vi "SP7_Kommunikation.vi"(8 "Fehler in":T1, 11 "Cluster in":T2={"Initialisierung"={"Online?"=FALSE, "Grundpfad"=path "", "Kamera Oben"="", "IP-Adresse Flüssiglinse"="", "Flüssiglinse"=refnum, "Kamera Unten"="", "IP-Adresse SPS"="", "SPS-Verbindung"={"TCP Connection Ref"=refnum, "IP address"="", "timeout ms"=5000, "Connected?"=FALSE, "PLC Type"=enum."S7 1200", "Rack S7 400"=0, "Slot S7 400"=0, "PDU Size"=0, "connection semaphore"=refnum}, "IP-Adresse Lichtgitter"="", "Lichtgitter"=refnum, "Skalierungsfaktor"=0.0, "Bilder Oben"=[], "Bild Unten"=refnum, "Bild Ausschnitt Unten"=refnum}, "Einstellungen"={"Gesamtablauf gestartet"=FALSE, "i. O. Bilder speichern"=FALSE, "Bildspeicherung Offline"=FALSE, "Ausgewähltes Offline-Datum"="", "Ausgewähltes Offline-Teil"="", "Speicherpfad Bilder"=path ""}, "Artikeldaten"={"Artikelnummer"="", "Fertigungsauftrag"="", "Muster ISO"=refnum, "Belichtungszeit Referenzmarken"=0.0, "Fokus Referenzmarken"=0.0, "Belichtungszeit ISO"=0.0, "Fokus ISO"=0.0, "Belichtungszeit Unten"=0.0, "Kontaktanzahl"=0, "Aktueller Kontakt"=0, "Kontaktposition"={"x"=0.0, "y"=0.0}, "Winkel ISO"=0.0, "ISO-Muster nicht vorhanden"=FALSE}, "Werte Kamera Oben"={"Koordinatensystem"={"Punkt x-Achse"={"X"=0.0, "Y"=0.0}, "Ursprung"={"X"=0.0, "Y"=0.0}, "Punkt y-Achse"={"X"=0.0, "Y"=0.0}}, "Position Kontakt"={"x"=0.0, "y"=0.0}, "Winkel Kontakt"=0.0}, "Werte Kamera Unten"={"Prüfung Unten n. i. O."=FALSE}, "Werte Lichtgitter"={"Messwerte Referenzmarken"=[], "Mittelpunkt Referenzmarken"={"x"=0.0, "y"=0.0}, "Messwerte Kontakt"=[], "Offset"={"x"=0.0, "y"=0.0}}, "Rückmeldungen"={"Koordinaten ermittelt"=FALSE, "Vermessung Lichtgitter fertig"=FALSE, "Nachkontrolle Kamera Unten fertig"=FALSE}, "Fehler"={"Referenzen nicht gefunden"=FALSE, "Kontakt nicht gefunden"=FALSE, "Referenzen nicht in Lichtgitter"=FALSE, "Kontakt zu groß"=FALSE, "Kontakt zu klein"=FALSE}, "Statistik"={"Statistiken"=[]}, "Timer"={"Timer Start Position"=0, "Timer Start Lichtgitter"=0, "Timer Start Kamera Unten"=0}}) -> (0 "error out":errorcluster)   [LabVIEW 2024]
doc: "Schreibt & liest alle Variablen der SPS."
uses:
  Cluster.ctl
  Kontaktmontagemodul.exe/1abvi3w/vi.lib/userDefined/High Color/IMAQdx.ctl
  Kontaktmontagemodul.exe/1abvi3w/vi.lib/DATA AHEAD/SP7/typedefs/S7 Connection.ctl
  Kontaktmontagemodul.exe/1abvi3w/vi.lib/DATA AHEAD/SP7/typedefs/PLC Type.ctl
  Kontaktmontagemodul.exe/1abvi3w/vi.lib/vision/Image Controls.llb/IMAQ Image.ctl
  Koordinatensystem.ctl
  Statistik.ctl
  Cluster_Fehler_Initialisierung.ctl
  Globale Variablen.vi
  Kontaktmontagemodul.exe/1abvi3w/vi.lib/DATA AHEAD/SP7/SP7.lvlib
panel:
  out "Druchlaufzeit (ms)":u32
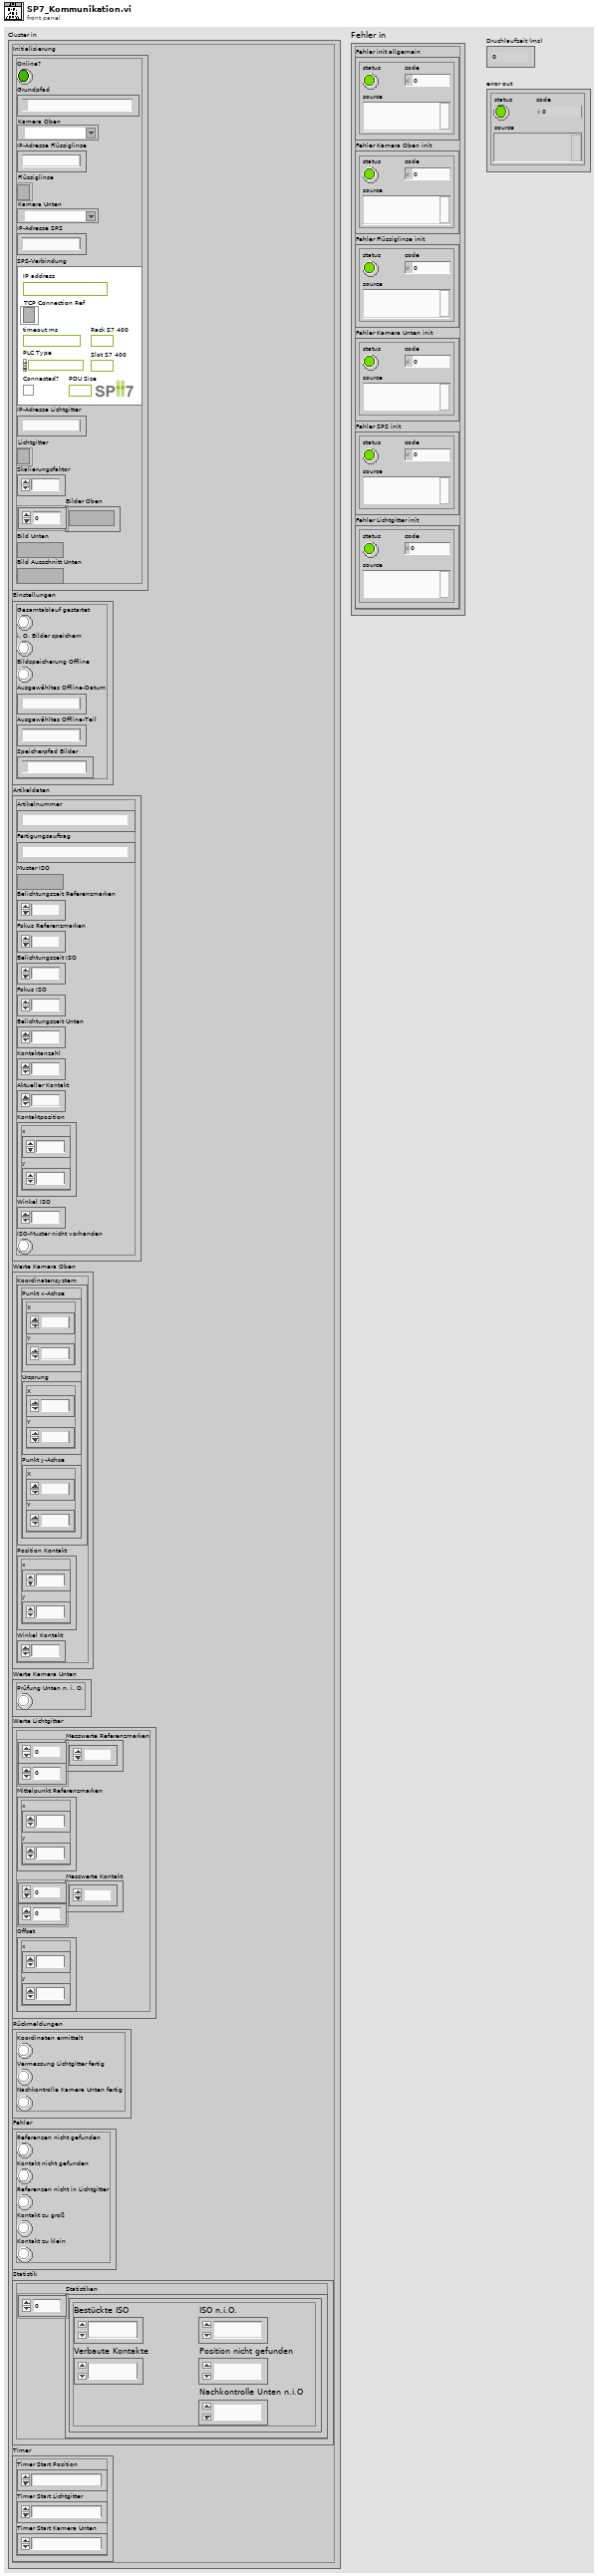
[diagram p1: front panel]
types:
  T1 = typedef "Cluster_Fehler_Initialisierung.ctl" = cluster{"Fehler init allgemein":errorcluster, "Fehler Kamera Oben init":errorcluster, "Fehler Flüssiglinse init":errorcluster, "Fehler Kamera Unten init":errorcluster, "Fehler SPS init":errorcluster, "Fehler Lichtgitter init":errorcluster}
  T2 = typedef "Cluster.ctl" = cluster{"Initialisierung":cluster{"Online?":bool, "Grundpfad":path, "Kamera Oben":T3, "IP-Adresse Flüssiglinse":string, "Flüssiglinse":refnum<k5>, "Kamera Unten":T3, "IP-Adresse SPS":string, "SPS-Verbindung":T4, "IP-Adresse Lichtgitter":string, "Lichtgitter":refnum<k5>, "Skalierungsfaktor":dbl, "Bilder Oben":T7[], "Bild Unten":T7, "Bild Ausschnitt Unten":T7}, "Einstellungen":cluster{"Gesamtablauf gestartet":bool, "i. O. Bilder speichern":bool, "Bildspeicherung Offline":bool, "Ausgewähltes Offline-Datum":string, "Ausgewähltes Offline-Teil":string, "Speicherpfad Bilder":path}, "Artikeldaten":cluster{"Artikelnummer":string, "Fertigungsauftrag":string, "Muster ISO":T7, "Belichtungszeit Referenzmarken":dbl, "Fokus Referenzmarken":dbl, "Belichtungszeit ISO":dbl, "Fokus ISO":dbl, "Belichtungszeit Unten":dbl, "Kontaktanzahl":u32, "Aktueller Kontakt":i16, "Kontaktposition":cluster{"x":sgl, "y":sgl}, "Winkel ISO":sgl, "ISO-Muster nicht vorhanden":bool}, "Werte Kamera Oben":cluster{"Koordinatensystem":T8, "Position Kontakt":cluster{"x":dbl, "y":dbl}, "Winkel Kontakt":dbl}, "Werte Kamera Unten":cluster{"Prüfung Unten n. i. O.":bool}, "Werte Lichtgitter":cluster{"Messwerte Referenzmarken":dbl[][], "Mittelpunkt Referenzmarken":cluster{"x":dbl, "y":dbl}, "Messwerte Kontakt":dbl[][], "Offset":cluster{"x":dbl, "y":dbl}}, "Rückmeldungen":cluster{"Koordinaten ermittelt":bool, "Vermessung Lichtgitter fertig":bool, "Nachkontrolle Kamera Unten fertig":bool}, "Fehler":cluster{"Referenzen nicht gefunden":bool, "Kontakt nicht gefunden":bool, "Referenzen nicht in Lichtgitter":bool, "Kontakt zu groß":bool, "Kontakt zu klein":bool}, "Statistik":cluster{"Statistiken":T9[]}, "Timer":cluster{"Timer Start Position":u32, "Timer Start Lichtgitter":u32, "Timer Start Kamera Unten":u32}}
  T3 = typedef "IMAQdx.ctl" = refnum<k21>
  T4 = typedef "SP7.lvlib/S7 Connection.ctl" = cluster{"TCP Connection Ref":refnum<k5>, "IP address":string, "timeout ms":i32, "Connected?":bool, "PLC Type":T5, "Rack S7 400":u8, "Slot S7 400":u8, "PDU Size":u16, "connection semaphore":T6}
  T5 = typedef "SP7.lvlib/PLC Type.ctl" = enum16{"S7 200", "S7 300/400", "S7 1200", "S7 1500", "LOGO!8"}
  T6 = typedef "Semaphore RefNum" = refnum<k1>
  T7 = typedef "IMAQ Image.ctl" = refnum<image>
  T8 = typedef "Koordinatensystem.ctl" = cluster{"Punkt x-Achse":cluster{"X":sgl, "Y":sgl}, "Ursprung":cluster{"X":sgl, "Y":sgl}, "Punkt y-Achse":cluster{"X":sgl, "Y":sgl}}
  T9 = typedef "Statistik.ctl" = cluster{"Bestückte ISO":u32, "Verbaute Kontakte":u32, "ISO n.i.O.":u32, "Nachkontrolle Unten n.i.O":u32, "Position nicht gefunden":u32}
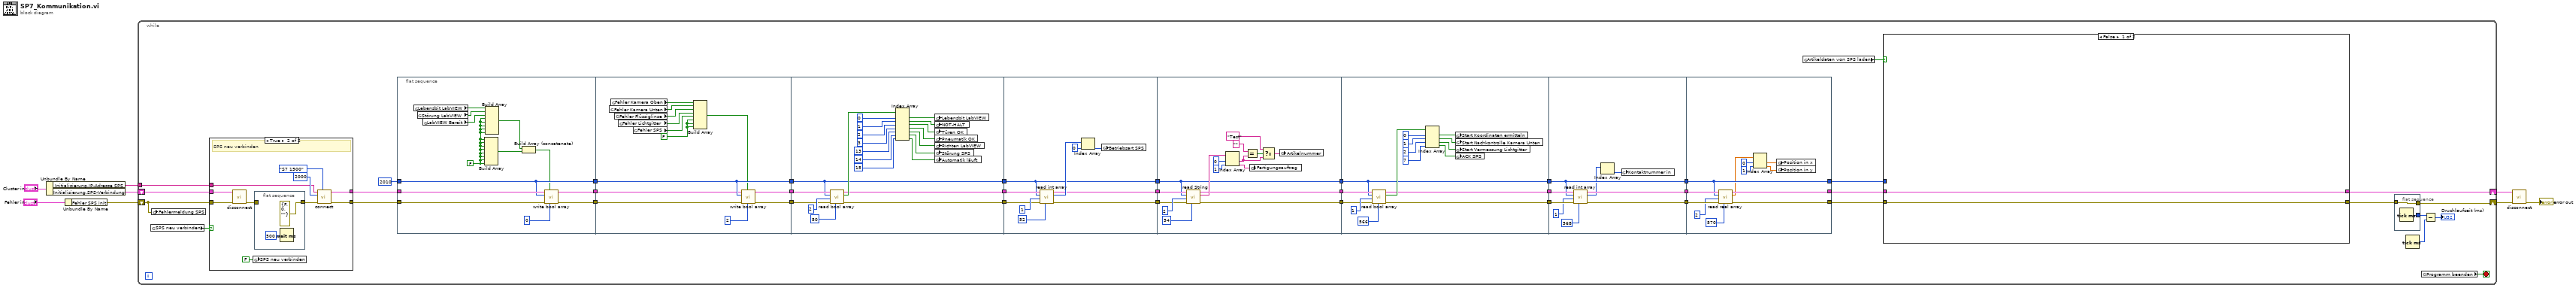
[diagram p0: block diagram]
diagram:
  n1 = Unbundle By Name("Cluster in") -> ("Initialisierung.IP-Adresse SPS"=w1:string, "Initialisierung.SPS-Verbindung"=w6:T4)
  n2 = Unbundle By Name("Fehler in") -> ("Fehler SPS init"=w3:errorcluster)
  n3 = while {
    shift-right: [w47] -> w8
    shift-left: w6 -> [w42]
    shift-right: [w39] -> w7
    shift-left: w3 -> [w41]
    tunnel: w1 -> [w40]
    stop <- w44 stop-if-true
    n4 = global read "Globale Variablen.vi" "SPS neu verbinden"() -> (w43:bool)
    n5 = global write "Globale Variablen.vi" "Fehlermeldung SPS"(w41) -> ()
    n6 = case shown="True" w43 {
      tunnel: w42 -> [w162 w171]
      tunnel: w41 -> [w161 w170]
      tunnel: [w161 w166] -> w35
      tunnel: [w162 w165] -> w34
      tunnel: w40 -> [_ w163]
      frame False {
      }
      frame True {
        # "SPS neu verbinden"
        n7 = call "disconnect.vi"("error in (no error)"=w170, "S7 Connection in"=w171) -> ("error out"=w169:errorcluster)  [unwired: 8 in, 1 out]
        n8 = global write "Globale Variablen.vi" "SPS neu verbinden"(FALSE ("SPS neu verbinden")) -> ()
        n9 = flat-sequence {
          tunnel: w169 -> [_]
          tunnel: [errorcluster {"status"=FALSE, "code"=0, "source"=""} ("error in (no error)")] -> w164
          frame #0 {
            n10 = Wait (ms)(milliseconds to wait=u32 500) -> ()  [unwired: 1 out]
          }
        }
        n11 = call "connect.vi"("PLC Type"=PLC_Type."S7 1500", "error in (no error)"=w164, "timeout [ms]"=2000, "IP address"=w163) -> ("error out"=w166:errorcluster, "S7 Connection out"=w165:T4)  [unwired: 6 in]
      }
    }
    n12 = flat-sequence {
      tunnel: w35 -> [w59]
      tunnel: w34 -> [w60]
      tunnel: u16 2010 ("Data Block #") -> [w58]
      tunnel: [w58] -> w33
      tunnel: [w54] -> w32
      tunnel: [w53] -> w31
      tunnel: w33 -> [w72]
      tunnel: w32 -> [w71]
      tunnel: w31 -> [w73]
      tunnel: [w72] -> w30
      tunnel: [w70] -> w29
      tunnel: [w69] -> w28
      tunnel: [w74] -> w26
      tunnel: [w75] -> w25
      tunnel: [w76] -> w19
      tunnel: w30 -> [w74]
      tunnel: w29 -> [w77]
      tunnel: w28 -> [w78]
      tunnel: w26 -> [w96]
      tunnel: w25 -> [w99]
      tunnel: [w98] -> w24
      tunnel: [w97] -> w23
      tunnel: w19 -> [w100]
      tunnel: [w96] -> w18
      tunnel: w24 -> [w115]
      tunnel: w23 -> [w113]
      tunnel: [w111] -> w22
      tunnel: [w114] -> w21
      tunnel: [w112] -> w20
      tunnel: w18 -> [w111]
      tunnel: w22 -> [w124]
      tunnel: w21 -> [w128]
      tunnel: w20 -> [w126]
      tunnel: [w124] -> w14
      tunnel: [w127] -> w13
      tunnel: [w125] -> w12
      tunnel: w14 -> [w142]
      tunnel: w13 -> [w146]
      tunnel: w12 -> [w145]
      tunnel: [w142] -> w11
      tunnel: [w144] -> w10
      tunnel: [w143] -> w9
      tunnel: [w157] -> w16
      tunnel: [w158] -> w17
      tunnel: [w153] -> w15
      tunnel: w11 -> [w153]
      tunnel: w10 -> [w155]
      tunnel: w9 -> [w156]
      frame #0 {
        w48 = FALSE
        n13 = global read "Globale Variablen.vi" "Lebensbit LabVIEW"() -> (w57:bool)
        n14 = global read "Globale Variablen.vi" "Störung LabVIEW"() -> (w56:bool)
        n15 = global read "Globale Variablen.vi" "LabVIEW Bereit"() -> (w55:bool)
        n16 = Build Array(w48, w48, w48, w48, w48, w48, w48, w48) -> (w51:bool[])
        n17 = Build Array(w57, w56, w55, w48, w48, w48, w48, w48) -> (w50:bool[])
        n18 = Build Array (concatenate)(w50, w51) -> (w49:bool[])
        n19 = call "write bool array.vi"("Item offset [byte]"=u32 0, "BOOL input array [byte]"=w49, "error in (no error)"=w59, "Data Block #"=w58, "S7 Connection in"=w60) -> ("error out"=w53:errorcluster, "S7 Connection out"=w54:T4)  [unwired: 3 in, 2 out]
      }
      frame #1 {
        w62 = FALSE
        n20 = global read "Globale Variablen.vi" "Fehler Kamera Unten"() -> (w66:bool)
        n21 = global read "Globale Variablen.vi" "Fehler Kamera Oben"() -> (w67:bool)
        n22 = global read "Globale Variablen.vi" "Fehler Flüssiglinse"() -> (w65:bool)
        n23 = global read "Globale Variablen.vi" "Fehler Lichtgitter"() -> (w64:bool)
        n24 = global read "Globale Variablen.vi" "Fehler SPS"() -> (w63:bool)
        n25 = Build Array(w67, w66, w65, w64, w63, w62, w62, w62) -> (w61:bool[])
        n26 = call "write bool array.vi"("Item offset [byte]"=u32 2, "BOOL input array [byte]"=w61, "error in (no error)"=w73, "Data Block #"=w72, "S7 Connection in"=w71) -> ("error out"=w69:errorcluster, "S7 Connection out"=w70:T4)  [unwired: 3 in, 2 out]
      }
      frame #2 {
        n27 = call "read bool array.vi"("Item offset [byte]"=u32 50, "error in (no error)"=w78, "Items # [byte]"=u16 2, "Data Block #"=w74, "S7 Connection in"=w77) -> ("error out"=w75:errorcluster, "BOOL result array  [byte]"=w88:bool[], "S7 Connection out"=w76:T4)  [unwired: 4 in]
        n28 = Index Array(array=w88, index #1=0 ("index"), index #2=1 ("index"), index #3=2 ("index"), index #4=3 ("index"), index #5=13 ("index"), index #6=14 ("index"), index #7=15 ("index")) -> (element #1=w89:bool, element #2=w91:bool, element #3=w90:bool, element #4=w92:bool, element #5=w95:bool, element #6=w94:bool, element #7=w93:bool)
        n29 = global write "Globale Variablen.vi" "Lebensbit LabVIEW"(w89) -> ()
        n30 = global write "Globale Variablen.vi" "NOT-HALT"(w91) -> ()
        n31 = global write "Globale Variablen.vi" "Türen OK"(w90) -> ()
        n32 = global write "Globale Variablen.vi" "Pneumatik OK"(w92) -> ()
        n33 = global write "Globale Variablen.vi" "Richten LabVIEW"(w95) -> ()
        n34 = global write "Globale Variablen.vi" "Störung SPS"(w94) -> ()
        n35 = global write "Globale Variablen.vi" "Automatik läuft"(w93) -> ()
      }
      frame #3 {
        n36 = call "read int array.vi"("Item offset [byte]"=u32 52, "error in (no error)"=w99, "items #"=u16 1, "Data Block #"=w96, "S7 Connection in"=w100) -> ("error out"=w98:errorcluster, "Int result array"=w104:i16[], "S7 Connection out"=w97:T4)  [unwired: 4 in]
        n37 = Index Array(array=w104, index=0) -> (element=w105:i16)
        n38 = global write "Globale Variablen.vi" "Betriebsart SPS"(w105) -> ()
      }
      frame #4 {
        n39 = call "read String.vi"("Item offset [byte]"=u32 54, "error in (no error)"=w115, "items #"=u16 2, "Data Block #"=w111, "S7 Connection in"=w113) -> ("error out"=w114:errorcluster, "STRING result Array"=w120:string[], "S7 Connection out"=w112:T4)  [unwired: 3 in, 1 out]
        n40 = Index Array(array=w120, index #1=0 ("index"), index #2=1 ("index")) -> (element #1=w107:string, element #2=w121:string)
        n41 = Equal?(x="", y=w107) -> (x = y?=w109:bool)
        n42 = global write "Globale Variablen.vi" "Fertigungsauftrag"(w121) -> ()
        n43 = Select(t="Test" ("Artikelnummer"), s=w109, f=w107) -> (s? t:f=w106:string)
        n44 = global write "Globale Variablen.vi" "Artikelnummer"(w106) -> ()
      }
      frame #5 {
        n45 = call "read bool array.vi"("Item offset [byte]"=u32 566, "error in (no error)"=w128, "Items # [byte]"=u16 1, "Data Block #"=w124, "S7 Connection in"=w126) -> ("error out"=w127:errorcluster, "BOOL result array  [byte]"=w134:bool[], "S7 Connection out"=w125:T4)  [unwired: 4 in]
        n46 = Index Array(array=w134, index #1=0 ("index"), index #2=1 ("index"), index #3=2 ("index"), index #4=7 ("index")) -> (element #1=w135:bool, element #2=w137:bool, element #3=w136:bool, element #4=w122:bool)
        n47 = global write "Globale Variablen.vi" "Start Koordinaten ermitteln"(w135) -> ()
        n48 = global write "Globale Variablen.vi" "Start Nachkontrolle Kamera Unten"(w137) -> ()
        n49 = global write "Globale Variablen.vi" "Start Vermessung Lichtgitter"(w136) -> ()
        n50 = global write "Globale Variablen.vi" "ACK SPS"(w122) -> ()
      }
      frame #6 {
        n51 = call "read int array.vi"("Item offset [byte]"=u32 568, "error in (no error)"=w146, "items #"=u16 1, "Data Block #"=w142, "S7 Connection in"=w145) -> ("error out"=w144:errorcluster, "Int result array"=w140:i16[], "S7 Connection out"=w143:T4)  [unwired: 4 in]
        n52 = Index Array(array=w140) -> (element=w139:i16)  [unwired: 1 in]
        n53 = global write "Globale Variablen.vi" "Kontaktnummer in"(w139) -> ()
      }
      frame #7 {
        n54 = call "read real array.vi"("Item offset [byte]"=u32 570, "error in (no error)"=w155, "items #"=u16 2, "Data Block #"=w153, "S7 Connection in"=w156) -> ("error out"=w158:errorcluster, "REAL result array"=w150:sgl[], "S7 Connection out"=w157:T4)  [unwired: 4 in]
        n55 = Index Array(array=w150, index #1=0 ("index"), index #2=1 ("index")) -> (element #1=w149:sgl, element #2=w148:sgl)
        n56 = global write "Globale Variablen.vi" "Position in x"(w149) -> ()
        n57 = global write "Globale Variablen.vi" "Position in y"(w148) -> ()
      }
    }
    n58 = global read "Globale Variablen.vi" "Artikeldaten von SPS laden"() -> (w37:bool)
    n59 = case shown="False" w37 {
      tunnel: [w176 w178] -> w47
      tunnel: w17 -> [w175 w177]
      tunnel: w16 -> [w176 w178]
      tunnel: [w175 w177] -> w27
      tunnel: w15 -> [_ _]
      frame False {
      }
      frame True {
        # "Die Artikeldaten werden nur bei Artikelwechsel geladen (spart Durchlaufzeit bei dieser Schleife, vielleicht auch vernachlässigbar)"
        n60 = global write "Globale Variablen.vi" "Artikeldaten von SPS laden"(FALSE ("Artikeldaten von SPS laden")) -> ()
      }
    }
    n61 = flat-sequence {
      tunnel: w27 -> [w160]
      tunnel: [w160] -> w39
      tunnel: [w159] -> w38
      frame #0 {
        n62 = Tick Count (ms)() -> (millisecond timer value=w159:u32)
      }
    }
    n63 = Tick Count (ms)() -> (millisecond timer value=w46:u32)
    n64 = global read "Globale Variablen.vi" "Programm beenden"() -> (w44:bool)
    n65 = Subtract(x=w38, y=w46) -> (x-y=→"Druchlaufzeit (ms)":u32)
  }
  n66 = call "disconnect.vi"("error in (no error)"=w7, "S7 Connection in"=w8) -> ("error out"=→"error out":errorcluster)  [unwired: 8 in, 1 out]
